vi "Number of Parameters.vi"(8 "error in (no error)":errorcluster, 11 "Parameterized Test Suite in":refnum<class "Parameterized Test Suite.lvclass">) -> (0 "error out":errorcluster, 2 "Number of Parameters":i32, 3 "Parameterized Test Suite out":refnum<class "Parameterized Test Suite.lvclass">)   [LabVIEW 2020]
uses:
  Parameterized Test Suite.lvclass
  C:/Program Files (x86)/National Instruments/LabVIEW 2020/vi.lib/Astemes/LUnit/Test Suite.lvclass
  <vilib>/Astemes/LUnit/Test Suite.lvclass
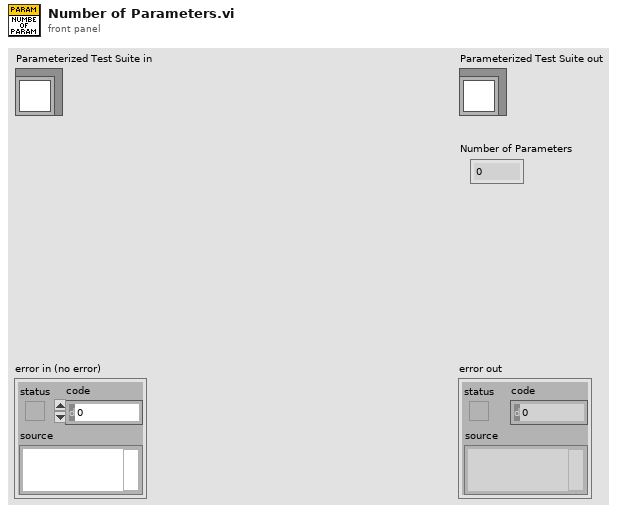
[diagram p1: front panel]
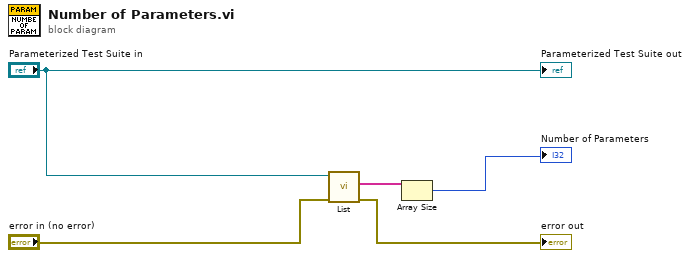
[diagram p0: block diagram]
diagram:
  n1 = call <vilib>:"List.vi"("error in (no error)"="error in (no error)", "LUnit Test Suite In"="Parameterized Test Suite in") -> ("error out"=→"error out":errorcluster, "List of Runnables"=w5:string[])  [unwired: 8 in]
  n2 = Array Size(array=w5) -> (size(s)=→"Number of Parameters":i32)
  "Parameterized Test Suite out" <- "Parameterized Test Suite in"
